vi "mcl_handle_error.vi"(8 "error in (no error)":errorcluster, 10 "No Error String":string, 11 "thorlabs_panel in":refnum<class "mcl_panel.lvclass">) -> (0 "error out":errorcluster, 3 "thorlabs_panel out":refnum<class "mcl_panel.lvclass">)   [LabVIEW 2015, in "mcl_panel.lvclass"]
uses:
  mcl_panel.lvclass
  mcl_panel.lvclass/mcl_panel.ctl
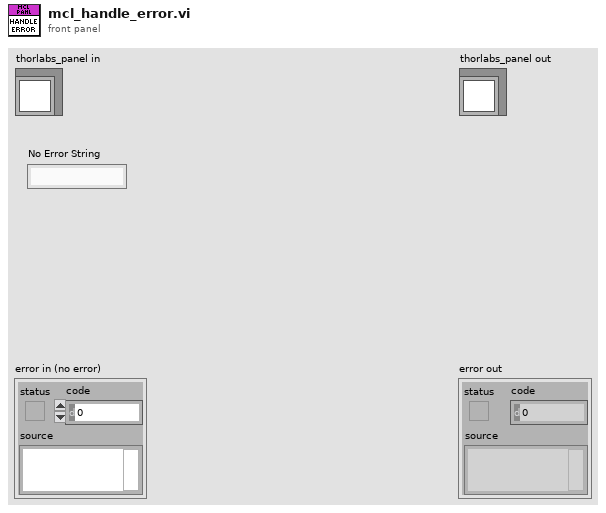
[diagram p1: front panel]
types:
  T1 = typedef "thorlabs_events.ctl" = cluster{"mcl_status":refnum<user-event>, "piezo_positions":refnum<user-event>}
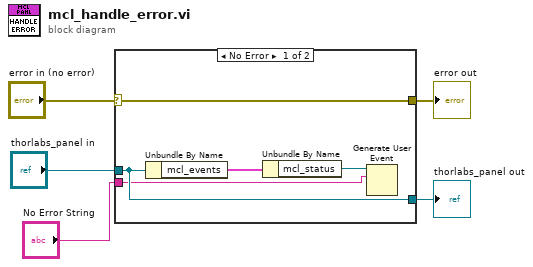
[diagram p0: block diagram]
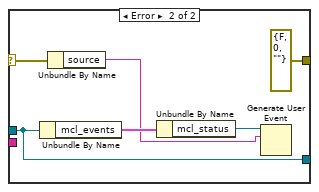
[diagram p2: hidden frame]
diagram:
  n1 = case shown="No Error" "error in (no error)" {
    selector: "error in (no error)" -> [w6 w16]
    tunnel: [w6 errorcluster {"status"=FALSE, "code"=0, "source"=""} ("error IO")] -> w4
    tunnel: [w8 w15] -> w2
    tunnel: "thorlabs_panel in" -> [w8 w15]
    tunnel: "No Error String" -> [w7 _]
    frame No Error {
      n2 = Unbundle By Name(w8) -> ("mcl_events"=w10:T1)
      n3 = Unbundle By Name(w10) -> ("mcl_status"=w9:refnum<user-event>)
      n4 = Generate User Event(user event=w9, event data cluster=w7) -> ()  [unwired: 2 in, 2 out]
    }
    frame Error {
      n5 = Unbundle By Name(w15) -> ("mcl_events"=w14:T1)
      n6 = Unbundle By Name(w16) -> ("source"=w12:string)
      n7 = Unbundle By Name(w14) -> ("mcl_status"=w13:refnum<user-event>)
      n8 = Generate User Event(user event=w13, event data cluster=w12) -> ()  [unwired: 2 in, 2 out]
    }
  }
  "error out" <- w4
  "thorlabs_panel out" <- w2
